vi "Validate.vi"() -> ()   [LabVIEW 2021, in "Online_SNR.lvclass"]
uses:
  Online_SNR.lvclass
  Online_SNR.lvclass/Online_SNR.ctl
panel:
  out "Error":dbl(graph)
  in  "noise":dbl
  out "SNR":dbl
  out "Signal":dbl(graph)
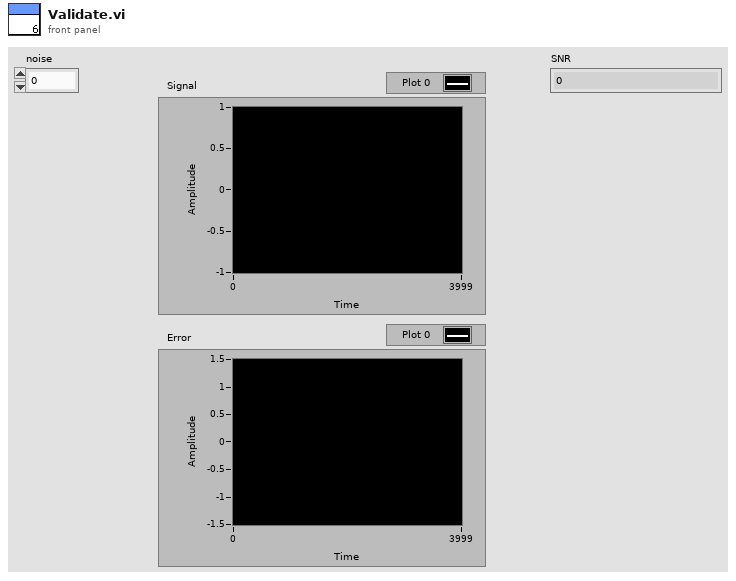
[diagram p1: front panel]
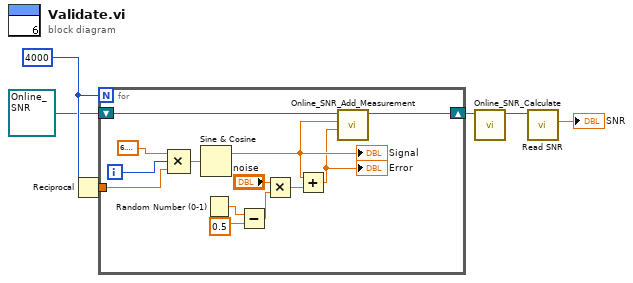
[diagram p0: block diagram]
diagram:
  w6 = 4000
  n1 = Reciprocal(x=w6) -> (1/x=w5:dbl)
  n2 = for {
    N: w6 -> [_]
    shift-right: [w14] -> w3
    shift-left: refnum<class "Online_SNR.lvclass"> refnum ("Online_SNR.lvclass") -> [w15]
    tunnel: w5 -> [w19]
    i -> [w18]
    n3 = Compound Arithmetic op=MULTIPLY(6.283185307179586, w18, w19) -> (w16:dbl)
    n4 = Sine & Cosine(0:w16) -> (1:w9:dbl)  [unwired: 1 out]
    "Signal" <- w9
    n5 = Random Number (0-1)() -> (number: 0 to 1=w12:dbl)
    n6 = Subtract(x=w12, y=0.5) -> (x-y=w11:dbl)
    n7 = Multiply(x="noise", y=w11) -> (x*y=w8:dbl)
    n8 = Add(x=w9, y=w8) -> (x+y=w7:dbl)
    "Error" <- w7
    n9 = call-dynamic "Online_SNR_Add_Measurement.vi"("Estimate"=w7, "True"=w9, "Online_SNR in"=w15) -> ("Online_SNR out"=w14:refnum<class "Online_SNR.lvclass">)  [unwired: 7 in, 1 out]
  }
  n10 = call "Online_SNR_Calculate.vi"("Online_SNR in"=w3) -> ("Online_SNR out"=w1:refnum<class "Online_SNR.lvclass">)  [unwired: 9 in, 1 out]
  n11 = call "Read SNR.vi"("Online_SNR in"=w1) -> ("SNR"=→"SNR":dbl)  [unwired: 8 in, 2 out]
